vi "SQL_创建表.vi"(6 "表名":string, 7 "数据库名":string, 8 "error in (no error)":errorcluster, 9 "列类型":string[](array[string]), 10 "列名":string[](array[string]), 11 "connection reference":T1) -> (0 "error out":errorcluster, 3 "connection reference 2":T1)   [LabVIEW 2014]
uses:
  <vilib>/addons/database/Connection.llb/Conn ObjectReference.ctl
  <vilib>/addons/database/Connection.llb/Conn Execute.vi
  <vilib>/addons/database/Recordset.llb/Rec Destroy - Connection.vi
  <vilib>/addons/database/NI_Database_API.lvlib
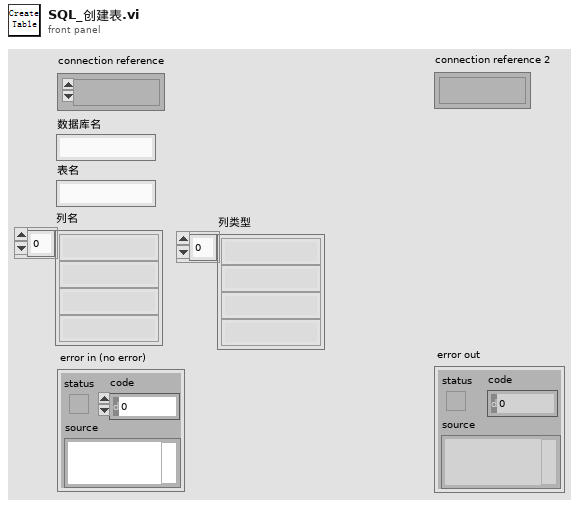
[diagram p1: front panel]
types:
  T1 = typedef "NI_Database_API.lvlib/Conn ObjectReference.ctl" = refnum<k1>
  T2 = typedef "NI_Database_API.lvlib/Rec ObjectReference.ctl" = refnum<k1>
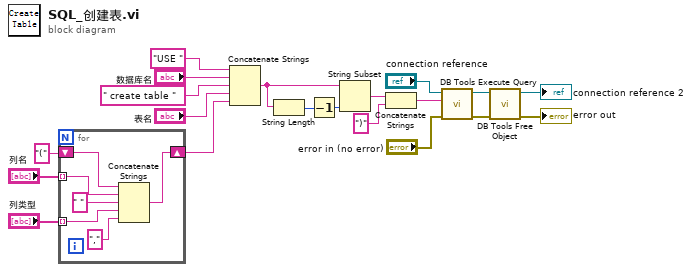
[diagram p0: block diagram]
diagram:
  n1 = for {
    tunnel: "列类型" -> [w23] mode=indexing
    tunnel: "列名" -> [w25] mode=indexing
    shift-right: [w22] -> w13
    shift-left: "(" -> [w26]
    n2 = Concatenate Strings(w26, w25, " " ("字符串"), w23, "," ("字符串")) -> (w22:string)
  }
  n3 = Concatenate Strings("USE " ("字符串"), "数据库名", " create table " ("字符串"), "表名", w13) -> (w12:string)
  n4 = String Length(string=w12) -> (length=w11:i32)
  n5 = Decrement(x=w11) -> (x-1=w10:i32)
  n6 = String Subset(string=w12, length (rest)=w10) -> (substring=w9:string)  [unwired: 1 in]
  n7 = Concatenate Strings(w9, ")" ("字符串")) -> (w4:string)
  n8 = call-poly <vilib>:"DB Tools Execute Query.vi"("error in (no error)"="error in (no error)", "SQL query"=w4, "connection reference"="connection reference") -> ("error out"=w5:errorcluster, "recordset reference"=w6:T2)  [unwired: 5 in]
  n9 = call-poly <vilib>:"DB Tools Free Object.vi"("error in (no error)"=w5, "recordset reference"=w6) -> ("error out"=→"error out":errorcluster, "connection reference"=→"connection reference 2":T1)  [unwired: 8 in]
